vi "Export multiple dat - tag.vi"(4 ".myDLTS file path":path, 5 "Error In":errorcluster, 6 "Workspace":path, 7 "Index":T1 {"IV"."IV properties"."Settling" min=0.0 max=65535.0; "CV"."CV properties"."V range" items=["10mV"=0.01, "100mV"=0.1, "1V"=1.0, "10V"=10.0]; "CV"."CV properties"."I range" items=["100nA"=-7.0, "1µA"=-6.0, "10µA"=-5.0, "100µA"=-4.0, "1mA"=-3.0, "10mA"=-2.0]; "LDLTS"."LDLTS properties"."V range" items=["10mV"=0.01, "100mV"=0.1, "1V"=1.0, "10V"=10.0]; "LDLTS"."LDLTS properties"."I range" items=["100nA"=-7.0, "1µA"=-6.0, "10µA"=-5.0, "100µA"=-4.0, "1mA"=-3.0, "10mA"=-2.0]; "Conv DLTS"."DLTS properties"."V range" items=["10mV"=0.01, "100mV"=0.1, "1V"=1.0, "10V"=10.0]; "Conv DLTS"."DLTS properties"."I range" items=["10mV"=0.01, "100mV"=0.1, "1V"=1.0, "10V"=10.0]}, 8 "Measurement tags":string[](array[string])) -> (0 "Error Out":errorcluster)   [LabVIEW 2019]
doc: "Handles export of measurement (identified by a tag) to a .dat file, displays a GUI window"
uses:
  Type defs/Session internal index Type Def.ctl
  Type defs/IV measurement Type Def.ctl
  Type defs/IV properties Type Def.ctl
  Type defs/CV measurement Type Def.ctl
  Type defs/CV properties Type Def.ctl
  Type defs/LDLTS measurement Type Def.ctl
  Type defs/LDLTS properties Type Def.ctl
  Type defs/cDLTS measurement Type Def.ctl
  Type defs/DLTS properties Type Def.ctl
  <vilib>/Utility/file.llb/Write Delimited Spreadsheet (string).vi
  <vilib>/Utility/file.llb/Write Delimited Spreadsheet (DBL).vi
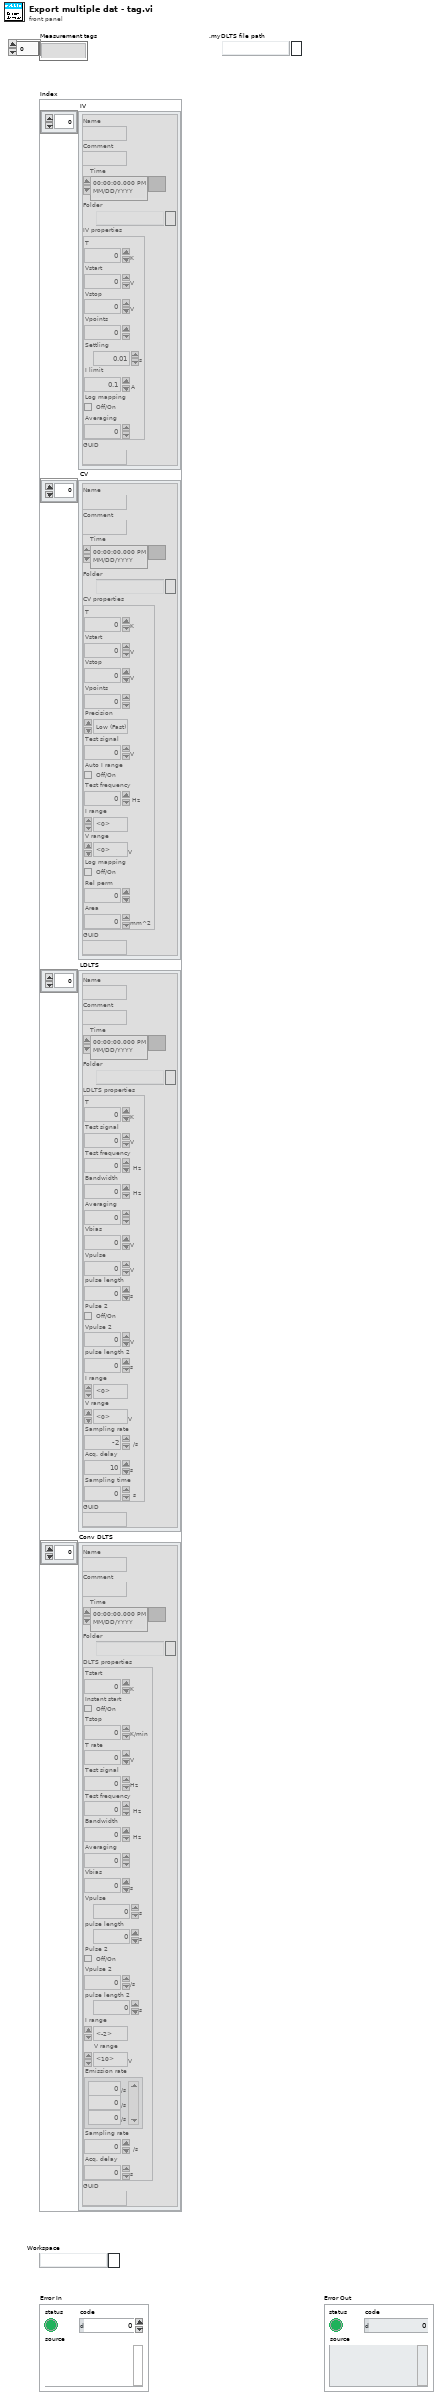
[diagram p1: front panel]
types:
  T1 = typedef "Session internal index Type Def.ctl" = cluster{"IV":T2[], "CV":T4[], "LDLTS":T6[], "Conv DLTS":T8[]}
  T2 = typedef "IV measurement Type Def.ctl" = cluster{"Name":string, "Comment":string, "Time":timestamp, "Folder":path, "IV properties":T3, "GUID":string}
  T3 = typedef "IV properties Type Def.ctl" = cluster{"T":dbl[unit], "Vstart":dbl[unit], "Vstop":dbl[unit], "Vpoints":dbl, "Settling":dbl[unit], "I limit":dbl[unit], "Log mapping":bool, "Averaging":dbl}
  T4 = typedef "CV measurement Type Def.ctl" = cluster{"Name":string, "Comment":string, "Time":timestamp, "Folder":path, "CV properties":T5, "GUID":string}
  T5 = typedef "CV properties Type Def.ctl" = cluster{"T":dbl[unit], "Vstart":dbl[unit], "Vstop":dbl[unit], "Vpoints":dbl, "Precision":enum16{"Low (Fast)", "Normal", "High (Slow)"}, "Test signal":dbl[unit], "Auto I range":bool, "Test frequency":dbl[unit], "I range":dbl, "V range":dbl[unit], "Log mapping":bool, "Rel perm":dbl, "Area":dbl[unit]}
  T6 = typedef "LDLTS measurement Type Def.ctl" = cluster{"Name":string, "Comment":string, "Time":timestamp, "Folder":path, "LDLTS properties":T7, "GUID":string}
  T7 = typedef "LDLTS properties Type Def.ctl" = cluster{"T":dbl[unit], "Test signal":dbl[unit], "Test frequency":dbl[unit], "Bandwidth":dbl[unit], "Averaging":dbl, "Vbias":dbl[unit], "Vpulse":dbl[unit], "pulse length":dbl[unit], "Pulse 2":bool, "Vpulse 2":dbl[unit], "pulse length 2":dbl[unit], "I range":dbl, "V range":dbl[unit], "Sampling rate":dbl[unit], "Acq. delay":dbl[unit], "Sampling time":dbl[unit]}
  T8 = typedef "cDLTS measurement Type Def.ctl" = cluster{"Name":string, "Comment":string, "Time":timestamp, "Folder":path, "DLTS properties":T9, "GUID":string}
  T9 = typedef "DLTS properties Type Def.ctl" = cluster{"Tstart":dbl[unit], "Instant start":bool, "Tstop":dbl[unit], "T rate":dbl[unit], "Test signal":dbl[unit], "Test frequency":dbl[unit], "Bandwidth":dbl[unit], "Averaging":dbl, "Vbias":dbl[unit], "Vpulse":dbl[unit], "pulse length":dbl[unit], "Pulse 2":bool, "Vpulse 2":dbl[unit], "pulse length 2":dbl[unit], "I range":dbl, "V range":dbl[unit], "Emission rate":dbl[unit][], "Sampling rate":dbl[unit], "Acq. delay":dbl[unit]}
  T10 = cluster{"Name":string, "Files":path[], "Header":string[][]}
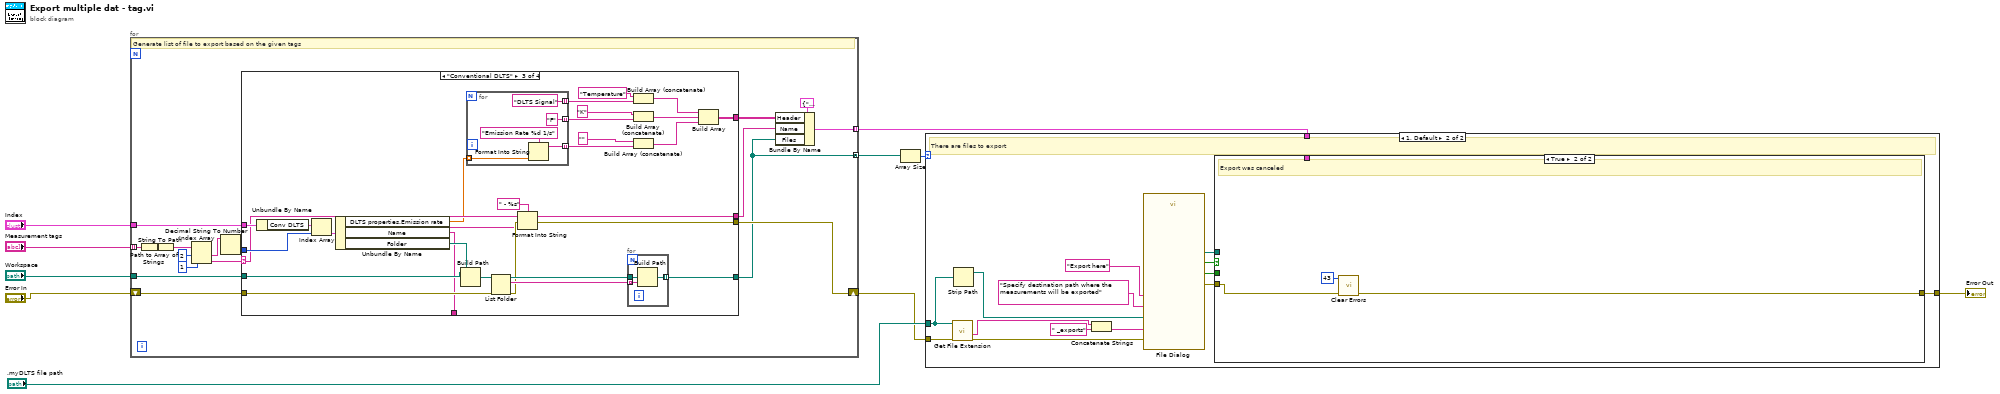
[diagram p0: block diagram]
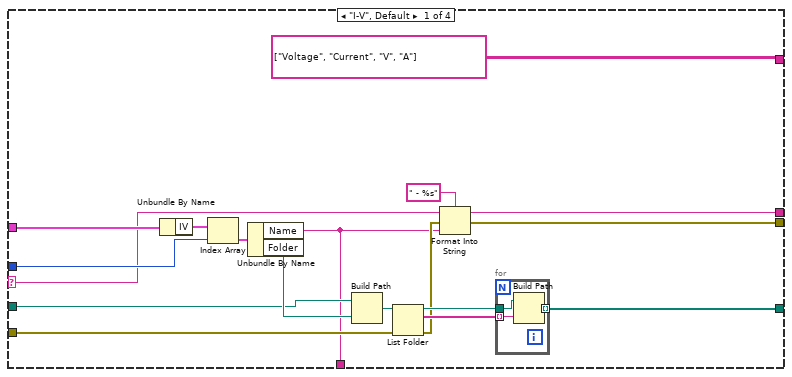
[diagram p2: hidden frame]
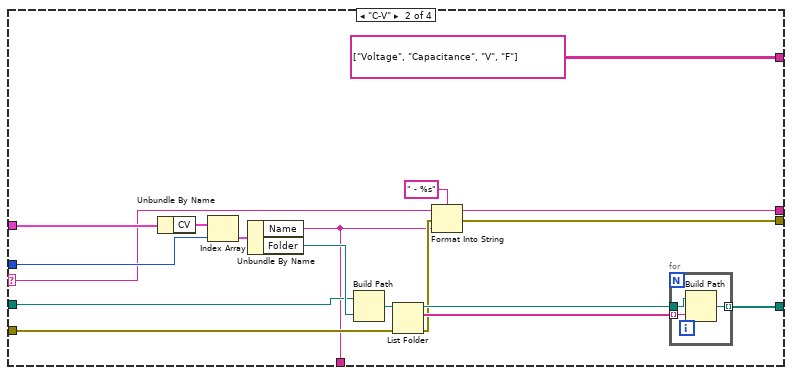
[diagram p3: hidden frame]
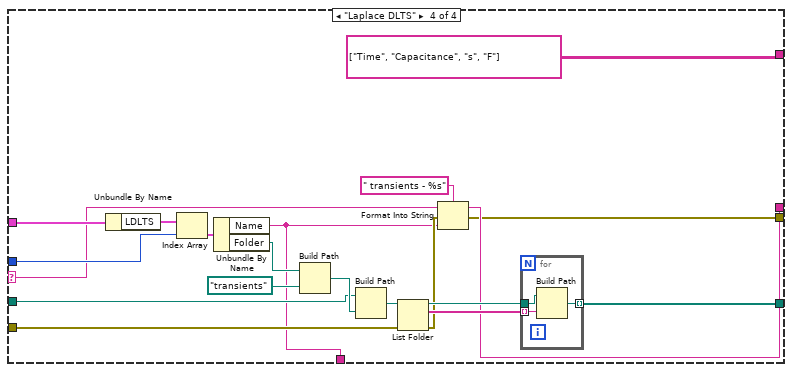
[diagram p4: hidden frame]
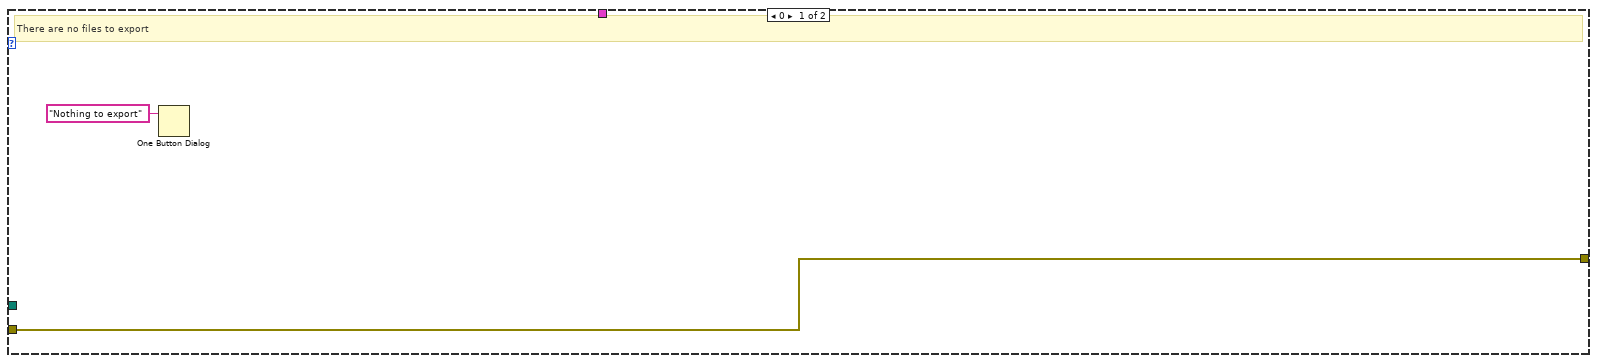
[diagram p5: hidden frame]
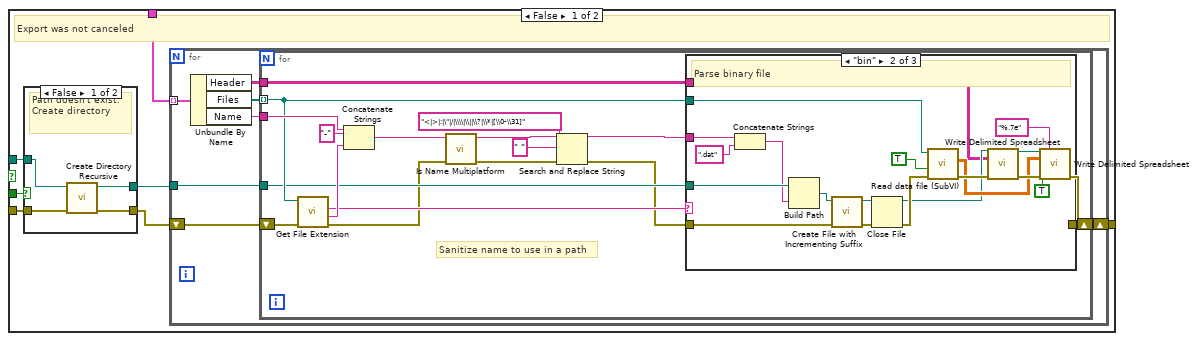
[diagram p6: hidden frame]
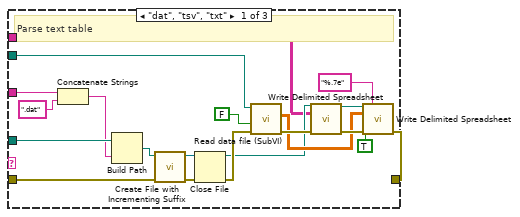
[diagram p7: hidden frame]
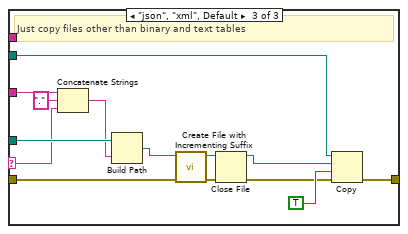
[diagram p8: hidden frame]
diagram:
  n1 = for {
    tunnel: "Measurement tags" -> [w23] mode=indexing
    tunnel: "Index" -> [w20]
    tunnel: "Workspace" -> [w18]
    tunnel: [w12] -> w6 mode=concatenating
    shift-right: [w17] -> w3
    shift-left: "Error In" -> [w16]
    tunnel: [w13] -> w2 mode=indexing
    # "Generate list of file to export based on the given tags"
    n2 = String To Path(string=w23) -> (path=w27:path)
    n3 = Path to Array of Strings(0:w27) -> (2:w26:string[])  [unwired: 1 out]
    n4 = Index Array(array=w26, index #1=2 ("index"), index #2=1 ("index")) -> (element #1=w21:string, element #2=w22:string)
    n5 = Decimal String To Number(string=w21) -> (number=w19:i32)  [unwired: 2 in, 1 out]
    n6 = case shown="\"Conventional DLTS\"" w22 {
      selector: w22 -> [w41 w62 w93 w121]
      tunnel: w20 -> [w45 w66 w97 w125]
      tunnel: w19 -> [w43 w64 w95 w123]
      tunnel: [w38 w59 w91 w119] -> w12
      tunnel: w16 -> [w36 w57 w89 w117]
      tunnel: [w28 w49 w70 w106] -> w17
      tunnel: w18 -> [w33 w54 w86 w112]
      tunnel: [w32 w52 w84 w109] -> w11
      tunnel: [string[][] [["Voltage", "Current"], ["V", "A"]] string[][] [["Voltage", "Capacitance"], ["V", "F"]] w72 string[][] [["Time", "Capacitance"], ["s", "F"]]] -> w14
      tunnel: [w29 w50 w71 w107] -> _
      frame "I-V", Default {
        n7 = Unbundle By Name(w45) -> ("IV"=w44:T2[])
        n8 = Index Array(array=w44, index=w43) -> (element=w42:T2)
        n9 = Unbundle By Name(w42) -> ("Name"=w29:string, "Folder"=w39:path)
        n10 = Build Path(base path=w33, name or relative path=w39) -> (appended path=w35:path)
        n11 = List Folder(path=w35, error in=w36) -> (path out=w34:path, filenames=w37:string[], error out=w31:errorcluster)  [unwired: 2 in, 1 out]
        n12 = Format Into String(format string=" - %s", initial string=w41, error in=w31, w29) -> (resulting string=w32:string, error out=w28:errorcluster)
        n13 = for {
          tunnel: w34 -> [w48]
          tunnel: [w47] -> w38 mode=indexing
          tunnel: w37 -> [w46] mode=indexing
          n14 = Build Path(base path=w48, name or relative path=w46) -> (appended path=w47:path)
        }
      }
      frame "C-V" {
        n15 = Unbundle By Name(w66) -> ("CV"=w65:T4[])
        n16 = Index Array(array=w65, index=w64) -> (element=w63:T4)
        n17 = Unbundle By Name(w63) -> ("Name"=w50:string, "Folder"=w60:path)
        n18 = Build Path(base path=w54, name or relative path=w60) -> (appended path=w56:path)
        n19 = List Folder(path=w56, error in=w57) -> (path out=w55:path, filenames=w58:string[], error out=w53:errorcluster)  [unwired: 2 in, 1 out]
        n20 = Format Into String(format string=" - %s", initial string=w62, error in=w53, w50) -> (resulting string=w52:string, error out=w49:errorcluster)
        n21 = for {
          tunnel: w55 -> [w69]
          tunnel: [w68] -> w59 mode=indexing
          tunnel: w58 -> [w67] mode=indexing
          n22 = Build Path(base path=w69, name or relative path=w67) -> (appended path=w68:path)
        }
      }
      frame "Conventional DLTS" {
        n23 = Unbundle By Name(w97) -> ("Conv DLTS"=w96:T8[])
        n24 = Index Array(array=w96, index=w95) -> (element=w94:T8)
        n25 = Unbundle By Name(w94) -> ("DLTS properties.Emission rate"=w73:dbl[unit][], "Name"=w71:string, "Folder"=w74:path)
        n26 = Build Path(base path=w86, name or relative path=w74) -> (appended path=w87:path)
        n27 = for {
          tunnel: w73 -> [w102] mode=indexing
          tunnel: [w100] -> w80 mode=indexing
          tunnel: ["DLTS Signal"] -> w78 mode=indexing
          tunnel: ["F"] -> w79 mode=indexing
          n28 = Format Into String(format string="Emission Rate %d 1/s", w102) -> (resulting string=w100:string)  [unwired: 2 in, 1 out]
        }
        n29 = List Folder(path=w87, error in=w89) -> (path out=w88:path, filenames=w90:string[], error out=w85:errorcluster)  [unwired: 2 in, 1 out]
        n30 = Format Into String(format string=" - %s", initial string=w93, error in=w85, w71) -> (resulting string=w84:string, error out=w70:errorcluster)
        n31 = for {
          tunnel: w88 -> [w105]
          tunnel: [w104] -> w91 mode=indexing
          tunnel: w90 -> [w103] mode=indexing
          n32 = Build Path(base path=w105, name or relative path=w103) -> (appended path=w104:path)
        }
        n33 = Build Array (concatenate)("Temperature", w78) -> (w75:string[])
        n34 = Build Array (concatenate)("K", w79) -> (w76:string[])
        n35 = Build Array (concatenate)("", w80) -> (w77:string[])
        n36 = Build Array(w75, w76, w77) -> (w72:string[][])
      }
      frame "Laplace DLTS" {
        n37 = Unbundle By Name(w125) -> ("LDLTS"=w124:T6[])
        n38 = Index Array(array=w124, index=w123) -> (element=w122:T6)
        n39 = Unbundle By Name(w122) -> ("Name"=w107:string, "Folder"=w115:path)
        n40 = Build Path(base path=w115, name or relative path=path "transients") -> (appended path=w113:path)
        n41 = Build Path(base path=w112, name or relative path=w113) -> (appended path=w116:path)
        n42 = List Folder(path=w116, error in=w117) -> (path out=w111:path, filenames=w118:string[], error out=w110:errorcluster)  [unwired: 2 in, 1 out]
        n43 = Format Into String(format string=" transients - %s", initial string=w121, error in=w110, w107) -> (resulting string=w109:string, error out=w106:errorcluster)
        n44 = for {
          tunnel: w111 -> [w128]
          tunnel: [w127] -> w119 mode=indexing
          tunnel: w118 -> [w126] mode=indexing
          n45 = Build Path(base path=w128, name or relative path=w126) -> (appended path=w127:path)
        }
      }
    }
    n46 = Bundle By Name(cluster=T10 {"Name"="", "Files"=[], "Header"=[]} ("output cluster"), "Header"=w14, "Name"=w11, "Files"=w12) -> (w13:T10)
  }
  n47 = Array Size(array=w6) -> (size(s)=w7:i32)
  n48 = case shown="1, Default" w7 {
    tunnel: ".myDLTS file path" -> [_ w138]
    tunnel: w3 -> [w129 w137]
    tunnel: [w129 w131] -> w1
    tunnel: w2 -> [_ w132]
    frame 0 {
      # "There are no files to export"
      n49 = One Button Dialog(message="Nothing to export") -> ()  [unwired: 1 in, 1 out]
    }
    frame 1, Default {
      # "There are files to export"
      n50 = call <vilib>:"Get File Extension.vi"("error in (no error)"=w137, "file"=w138) -> ("error out"=w142:errorcluster, "filename without extension"=w144:string)  [unwired: 5 in, 3 out]
      n51 = Strip Path(path=w138) -> (stripped path=w143:path)  [unwired: 1 out]
      n52 = Concatenate Strings(w144, " _exports" ("string")) -> (w145:string)
      n53 = call "File Dialog"("start path"=w143, "prompt"="Specify destination path where the measurements will be exported", "button label"="Export here", "default name"=w145, "error in"=w142) -> ("selected path"=w133:path, "exists"=w135:bool, "cancelled"=w136:bool, "error out"=w134:errorcluster)  [unwired: 7 in]
      n54 = case shown="True" w136 {
        tunnel: w135 -> [w152 _]
        tunnel: w134 -> [w151 w239]
        tunnel: w133 -> [w150 _]
        tunnel: w132 -> [w147 _]
        tunnel: [w146 w238] -> w131
        frame False {
          # "Export was not canceled"
          n55 = case shown="False" w152 {
            tunnel: w151 -> [w234 w236]
            tunnel: w150 -> [w233 w235]
            tunnel: [w232 w235] -> w149
            tunnel: [w231 w236] -> w148
            frame False {
              # "Path doesn't exist.\nCreate directory"
              n56 = call <vilib>:"Create Directory Recursive.vi"("error in (no error)"=w234, "directory"=w233) -> ("error out"=w231:errorcluster, "directory copy"=w232:path)  [unwired: 3 in, 1 out]
            }
            frame True {
              # "Path exists"
            }
          }
          n57 = for {
            tunnel: w147 -> [w159] mode=indexing
            shift-right: [w154] -> w146
            shift-left: w148 -> [w155]
            tunnel: w149 -> [w153]
            n58 = Unbundle By Name(w159) -> ("Header"=w156:string[][], "Files"=w158:path[], "Name"=w157:string)
            n59 = for {
              tunnel: w158 -> [w170] mode=indexing
              tunnel: w157 -> [w175]
              tunnel: w156 -> [w169]
              shift-right: [w171] -> w154
              shift-left: w155 -> [w176]
              tunnel: w153 -> [w168]
              # "Sanitize name to use in a path"
              n60 = call <vilib>:"Get File Extension.vi"("error in (no error)"=w176, "file"=w170) -> ("error out"=w166:errorcluster, "filename without extension"=w173:string, "lowercase file extension"=w172:string)  [unwired: 5 in, 2 out]
              n61 = Concatenate Strings(w175, "-" ("string"), w173) -> (w167:string)
              n62 = call <vilib>:"Is Name Multiplatform.vi"("error in (no error)"=w166, "filename"=w167) -> ("error out"=w162:errorcluster, "suggested filename"=w161:string)  [unwired: 5 in, 3 out]
              n63 = Search and Replace String(input string=w161, search string="<|>|:|\"|/|\\\\|\\||\\?|\\*|[\\0-\\31]", replace string=" " ("replace string (\"\")"), error in=w162) -> (result string=w160:string, error out=w163:errorcluster)  [unwired: 4 in, 2 out]
              n64 = case shown="\"bin\"" w172 {
                selector: w172 -> [_ _ w222]
                tunnel: w160 -> [w196 w216 w230]
                tunnel: w163 -> [w184 w204 w227]
                tunnel: [w183 w203 w217] -> w171
                tunnel: w170 -> [w181 w201 w221]
                tunnel: w169 -> [w182 w202 _]
                tunnel: w168 -> [w179 w199 w226]
                frame "dat", "tsv", "txt" {
                  # "Parse text table"
                  n65 = Concatenate Strings(w196, ".dat" ("string")) -> (w178:string)
                  n66 = Build Path(base path=w179, name or relative path=w178) -> (appended path=w177:path)
                  n67 = call <vilib>:"Create File with Incrementing Suffix.vi"("error in (no error)"=w184, "file path"=w177) -> ("error out"=w188:errorcluster, "refnum out"=w187:refnum<file>)  [unwired: 7 in, 1 out]
                  n68 = Close File(refnum=w187, error in=w188) -> (path=w185:path, error out=w186:errorcluster)
                  n69 = call "Read data file (SubVI).vi"("error in"=w186, "Binary"=FALSE, "file path in"=w181) -> ("error out"=w190:errorcluster, "2D data"=w189:dbl[][])  [unwired: 6 in, 1 out]
                  n70 = call-poly <vilib>:"Write Delimited Spreadsheet.vi"("file path (dialog if empty)"=w185, "2D data"=w182, "error in (no error)"=w190) -> ("new file path (Not A Path if cancelled)"=w191:path, "error out"=w193:errorcluster)  [unwired: 11 in]
                  n71 = call-poly <vilib>:"Write Delimited Spreadsheet.vi"("file path (dialog if empty)"=w191, "format (%.3f)"="%.7e", "2D data"=w189, "append to file? (new file:F)"=TRUE, "error in (no error)"=w193) -> ("error out"=w183:errorcluster)  [unwired: 9 in, 1 out]
                }
                frame "bin" {
                  # "Parse binary file"
                  n72 = Concatenate Strings(w216, ".dat" ("string")) -> (w198:string)
                  n73 = Build Path(base path=w199, name or relative path=w198) -> (appended path=w197:path)
                  n74 = call <vilib>:"Create File with Incrementing Suffix.vi"("error in (no error)"=w204, "file path"=w197) -> ("error out"=w208:errorcluster, "refnum out"=w207:refnum<file>)  [unwired: 7 in, 1 out]
                  n75 = Close File(refnum=w207, error in=w208) -> (path=w205:path, error out=w206:errorcluster)
                  n76 = call "Read data file (SubVI).vi"("error in"=w206, "Binary"=TRUE, "file path in"=w201) -> ("error out"=w210:errorcluster, "2D data"=w209:dbl[][])  [unwired: 6 in, 1 out]
                  n77 = call-poly <vilib>:"Write Delimited Spreadsheet.vi"("file path (dialog if empty)"=w205, "2D data"=w202, "error in (no error)"=w210) -> ("new file path (Not A Path if cancelled)"=w211:path, "error out"=w213:errorcluster)  [unwired: 11 in]
                  n78 = call-poly <vilib>:"Write Delimited Spreadsheet.vi"("file path (dialog if empty)"=w211, "format (%.3f)"="%.7e", "2D data"=w209, "append to file? (new file:F)"=TRUE, "error in (no error)"=w213) -> ("error out"=w203:errorcluster)  [unwired: 9 in, 1 out]
                }
                frame "json", "xml", Default {
                  # "Just copy files other than binary and text tables"
                  n79 = Concatenate Strings(w230, "." ("string"), w222) -> (w225:string)
                  n80 = Build Path(base path=w226, name or relative path=w225) -> (appended path=w224:path)
                  n81 = call <vilib>:"Create File with Incrementing Suffix.vi"("error in (no error)"=w227, "file path"=w224) -> ("error out"=w229:errorcluster, "refnum out"=w228:refnum<file>)  [unwired: 7 in, 1 out]
                  n82 = Close File(refnum=w228, error in=w229) -> (path=w218:path, error out=w219:errorcluster)
                  n83 = Copy(8:w219, 9:TRUE ("overwrite (F)"), 10:w218, 11:w221) -> (0:w217:errorcluster)  [unwired: 1 in, 2 out]
                }
              }
            }
          }
        }
        frame True {
          # "Export was canceled"
          n84 = call <vilib>:"Clear Errors.vi"("error in (no error)"=w239, "specific error code to clear (0: all)"=43) -> ("error out"=w238:errorcluster)  [unwired: 4 in, 1 out]
        }
      }
    }
  }
  "Error Out" <- w1
